vi "Odległośc pomiędzy wybranymi robotami.vi"(9 "Lokalizacja robotów in":T1, 10 "Wybór robota 2":T2 items=["Łazik", "Quadron", "Dron 1", "Dron 2"], 11 "Wybór robota in":T2 items=["Łazik", "Quadron", "Dron 1", "Dron 2"]) -> (1 "Odległość pomiędzy\n robotami [m]":dbl, 2 "Odległości pomiędzy wybranymi robotami xy [m]":cluster{"X [m]":dbl, "Y [m]":dbl})   [LabVIEW 2015, in "Biblioteka moduł map v3.lvlib" / "Pomocnicze.lvlib"]
uses:
  Pomocnicze.lvlib
  Matematyczne/Matematyczne.lvlib
  Kontrolki/Kontrolki.lvlib
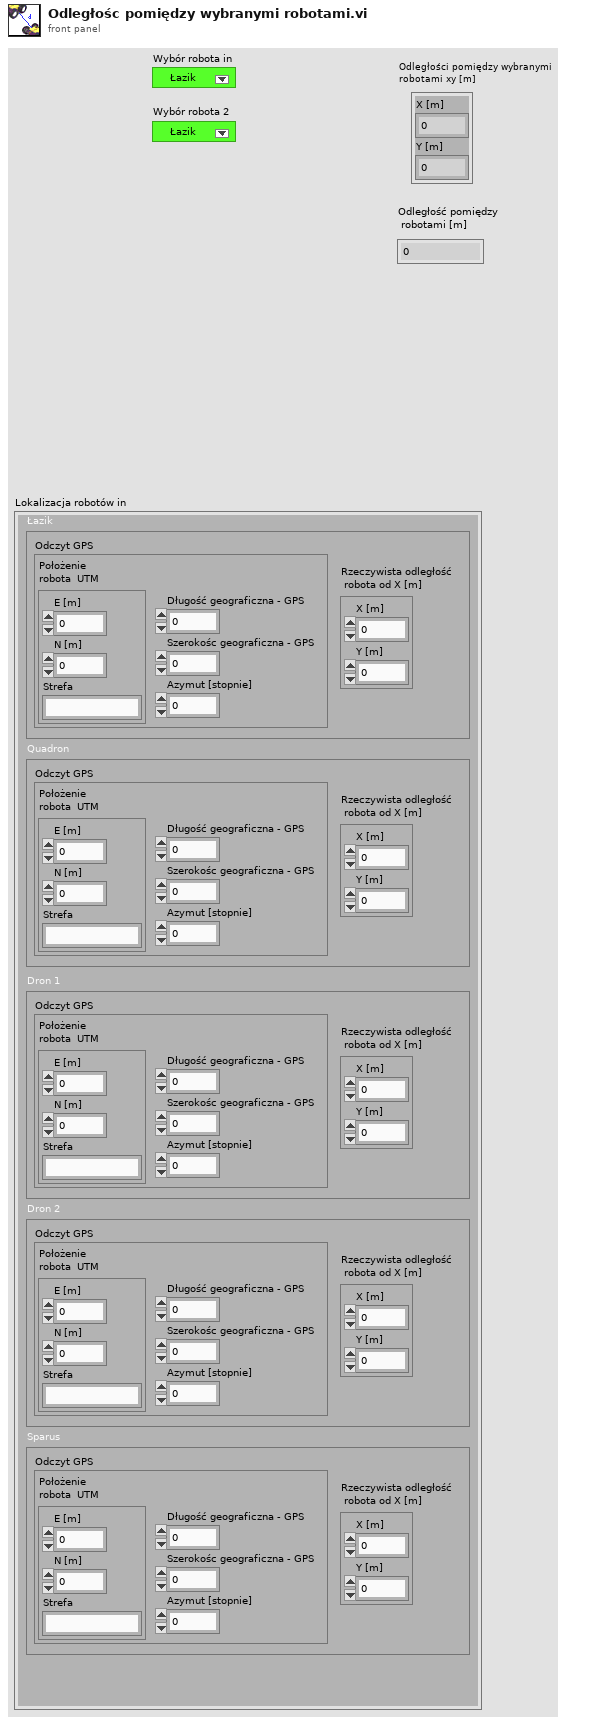
[diagram p1: front panel]
types:
  T1 = typedef "Biblioteka moduł map v3.lvlib/Kontrolki.lvlib/Lokalizacja robotów.ctl" = cluster{"Łazik":cluster{"Odczyt GPS":cluster{"Położenie \nrobota  UTM":cluster{"E [m]":ext, "N [m]":ext, "Strefa":string}, "Długość geograficzna - GPS":dbl, "Szerokośc geograficzna - GPS":dbl, "Azymut [stopnie]":dbl}, "Rzeczywista odległość\n robota od X [m]":cluster{"X [m]":dbl, "Y [m]":dbl}}, "Quadron":cluster{"Odczyt GPS":cluster{"Położenie \nrobota  UTM":cluster{"E [m]":ext, "N [m]":ext, "Strefa":string}, "Długość geograficzna - GPS":dbl, "Szerokośc geograficzna - GPS":dbl, "Azymut [stopnie]":dbl}, "Rzeczywista odległość\n robota od X [m]":cluster{"X [m]":dbl, "Y [m]":dbl}}, "Dron 1":cluster{"Odczyt GPS":cluster{"Położenie \nrobota  UTM":cluster{"E [m]":ext, "N [m]":ext, "Strefa":string}, "Długość geograficzna - GPS":dbl, "Szerokośc geograficzna - GPS":dbl, "Azymut [stopnie]":dbl}, "Rzeczywista odległość\n robota od X [m]":cluster{"X [m]":dbl, "Y [m]":dbl}}, "Dron 2":cluster{"Odczyt GPS":cluster{"Położenie \nrobota  UTM":cluster{"E [m]":ext, "N [m]":ext, "Strefa":string}, "Długość geograficzna - GPS":dbl, "Szerokośc geograficzna - GPS":dbl, "Azymut [stopnie]":dbl}, "Rzeczywista odległość\n robota od X [m]":cluster{"X [m]":dbl, "Y [m]":dbl}}, "Sparus":cluster{"Odczyt GPS":cluster{"Położenie \nrobota  UTM":cluster{"E [m]":ext, "N [m]":ext, "Strefa":string}, "Długość geograficzna - GPS":dbl, "Szerokośc geograficzna - GPS":dbl, "Azymut [stopnie]":dbl}, "Rzeczywista odległość\n robota od X [m]":cluster{"X [m]":dbl, "Y [m]":dbl}}}
  T2 = typedef "Biblioteka moduł map v3.lvlib/Kontrolki.lvlib/Wybór robota.ctl" = u16
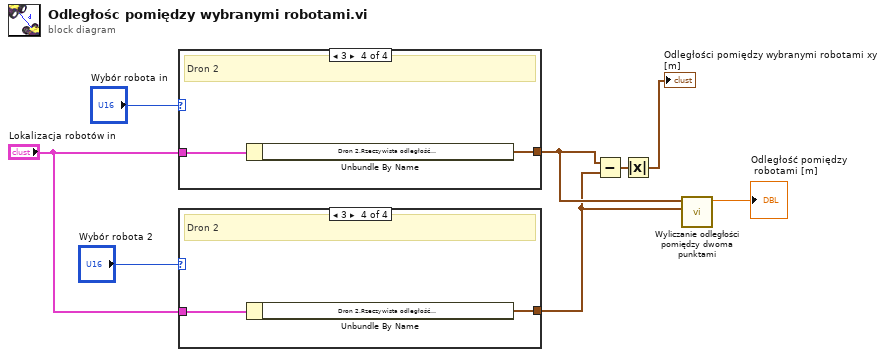
[diagram p0: block diagram]
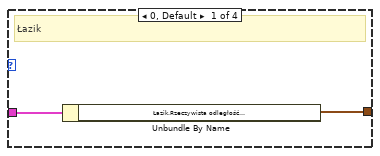
[diagram p2: hidden frame]
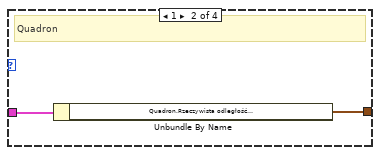
[diagram p3: hidden frame]
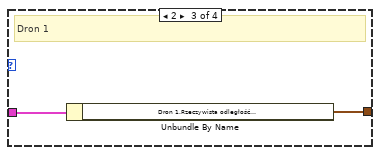
[diagram p4: hidden frame]
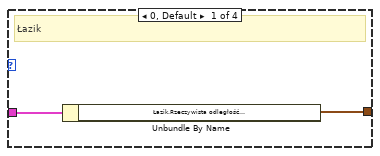
[diagram p5: hidden frame]
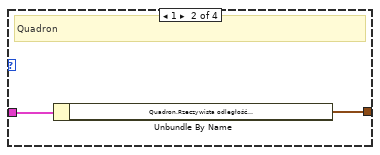
[diagram p6: hidden frame]
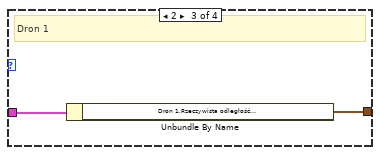
[diagram p7: hidden frame]
diagram:
  n1 = case shown="3" "Wybór robota in" {
    tunnel: "Lokalizacja robotów in" -> [w10 w12 w14 w16]
    tunnel: [w9 w11 w13 w15] -> w2
    frame 0, Default {
      # "Łazik"
      n2 = Unbundle By Name(w10) -> ("Łazik.Rzeczywista odległość\n robota od X [m]"=w9:cluster{"X [m]":dbl, "Y [m]":dbl})
    }
    frame 1 {
      # "Quadron"
      n3 = Unbundle By Name(w12) -> ("Quadron.Rzeczywista odległość\n robota od X [m]"=w11:cluster{"X [m]":dbl, "Y [m]":dbl})
    }
    frame 2 {
      # "Dron 1"
      n4 = Unbundle By Name(w14) -> ("Dron 1.Rzeczywista odległość\n robota od X [m]"=w13:cluster{"X [m]":dbl, "Y [m]":dbl})
    }
    frame 3 {
      # "Dron 2"
      n5 = Unbundle By Name(w16) -> ("Dron 2.Rzeczywista odległość\n robota od X [m]"=w15:cluster{"X [m]":dbl, "Y [m]":dbl})
    }
  }
  n6 = case shown="3" "Wybór robota 2" {
    tunnel: "Lokalizacja robotów in" -> [w18 w20 w22 w24]
    tunnel: [w17 w19 w21 w23] -> w1
    frame 0, Default {
      # "Łazik"
      n7 = Unbundle By Name(w18) -> ("Łazik.Rzeczywista odległość\n robota od X [m]"=w17:cluster{"X [m]":dbl, "Y [m]":dbl})
    }
    frame 1 {
      # "Quadron"
      n8 = Unbundle By Name(w20) -> ("Quadron.Rzeczywista odległość\n robota od X [m]"=w19:cluster{"X [m]":dbl, "Y [m]":dbl})
    }
    frame 2 {
      # "Dron 1"
      n9 = Unbundle By Name(w22) -> ("Dron 1.Rzeczywista odległość\n robota od X [m]"=w21:cluster{"X [m]":dbl, "Y [m]":dbl})
    }
    frame 3 {
      # "Dron 2"
      n10 = Unbundle By Name(w24) -> ("Dron 2.Rzeczywista odległość\n robota od X [m]"=w23:cluster{"X [m]":dbl, "Y [m]":dbl})
    }
  }
  n11 = Subtract(x=w2, y=w1) -> (x-y=w4:cluster{"X [m]":dbl, "Y [m]":dbl})
  n12 = Absolute Value(x=w4) -> (abs(x)=→"Odległości pomiędzy wybranymi robotami xy [m]":cluster{"X [m]":dbl, "Y [m]":dbl})
  n13 = call "Wyliczanie odległości pomiędzy dwoma punktami.vi"("Polozenie 1"=w1, "Polozenie in"=w2) -> ("Numeric"=→"Odległość pomiędzy\n robotami [m]":dbl)  [unwired: 9 in]
